vi "PicoScope6000aAdvancedTriggerDigital.vi"(0 "handle in":i16=16384, 2 "Digital Ports":T1 {"Digital Port  1"."Direction Channel 15" items=["Don't Care", "Low", "High", "Rising", "Falling"]; "Digital Port  1"."Direction Channel 14" items=["Don't Care", "Low", "High", "Rising", "Falling"]; "Digital Port  1"."Direction Channel 13" items=["Don't Care", "Low", "High", "Rising", "Falling"]; "Digital Port  1"."Direction Channel 12" items=["Don't Care", "Low", "High", "Rising", "Falling"]; "Digital Port  1"."Direction Channel 11" items=["Don't Care", "Low", "High", "Rising", "Falling"]; "Digital Port  1"."Direction Channel 10" items=["Don't Care", "Low", "High", "Rising", "Falling"]; "Digital Port  1"."Direction Channel 9" items=["Don't Care", "Low", "High", "Rising", "Falling"]; "Digital Port  1"."Direction Channel 8" items=["Don't Care", "Low", "High", "Rising", "Falling"]; "Digital Port  0"."Direction Channel 7" items=["Don't Care", "Low", "High", "Rising", "Falling"]; "Digital Port  0"."Direction Channel 6" items=["Don't Care", "Low", "High", "Rising", "Falling"]; "Digital Port  0"."Direction Channel 5" items=["Don't Care", "Low", "High", "Rising", "Falling"]; "Digital Port  0"."Direction Channel 4" items=["Don't Care", "Low", "High", "Rising", "Falling"]; "Digital Port  0"."Direction Channel 3" items=["Don't Care", "Low", "High", "Rising", "Falling"]; "Digital Port  0"."Direction Channel 2" items=["Don't Care", "Low", "High", "Rising", "Falling"]; "Digital Port  0"."Direction Channel 1" items=["Don't Care", "Low", "High", "Rising", "Falling"]; "Digital Port  0"."Direction Channel 0" items=["Don't Care", "Low", "High", "Rising", "Falling"]}, 11 "error in":errorcluster) -> (4 "handle out":i16=16384, 15 "error out":errorcluster)   [LabVIEW 2010]
doc: "This sub VI is an interface for the advanced trigger features of the oscilloscope to support digital channels."
uses:
  ps6000a.dll
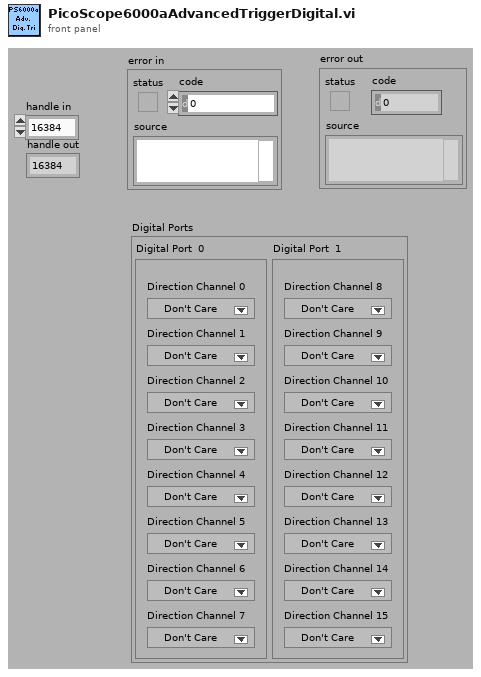
[diagram p1: front panel]
types:
  T1 = cluster{"Digital Port  0":cluster{"Direction Channel 0":u16, "Direction Channel 1":u16, "Direction Channel 2":u16, "Direction Channel 3":u16, "Direction Channel 4":u16, "Direction Channel 5":u16, "Direction Channel 6":u16, "Direction Channel 7":u16}, "Digital Port  1":cluster{"Direction Channel 8":u16, "Direction Channel 9":u16, "Direction Channel 10":u16, "Direction Channel 11":u16, "Direction Channel 12":u16, "Direction Channel 13":u16, "Direction Channel 14":u16, "Direction Channel 15":u16}}
  T2 = cluster{"Direction Channel 0":u16, "Direction Channel 1":u16, "Direction Channel 2":u16, "Direction Channel 3":u16, "Direction Channel 4":u16, "Direction Channel 5":u16, "Direction Channel 6":u16, "Direction Channel 7":u16}
  T3 = cluster{"Direction Channel 8":u16, "Direction Channel 9":u16, "Direction Channel 10":u16, "Direction Channel 11":u16, "Direction Channel 12":u16, "Direction Channel 13":u16, "Direction Channel 14":u16, "Direction Channel 15":u16}
  T4 = cluster{"status":bool, "code":u32, "source":string}
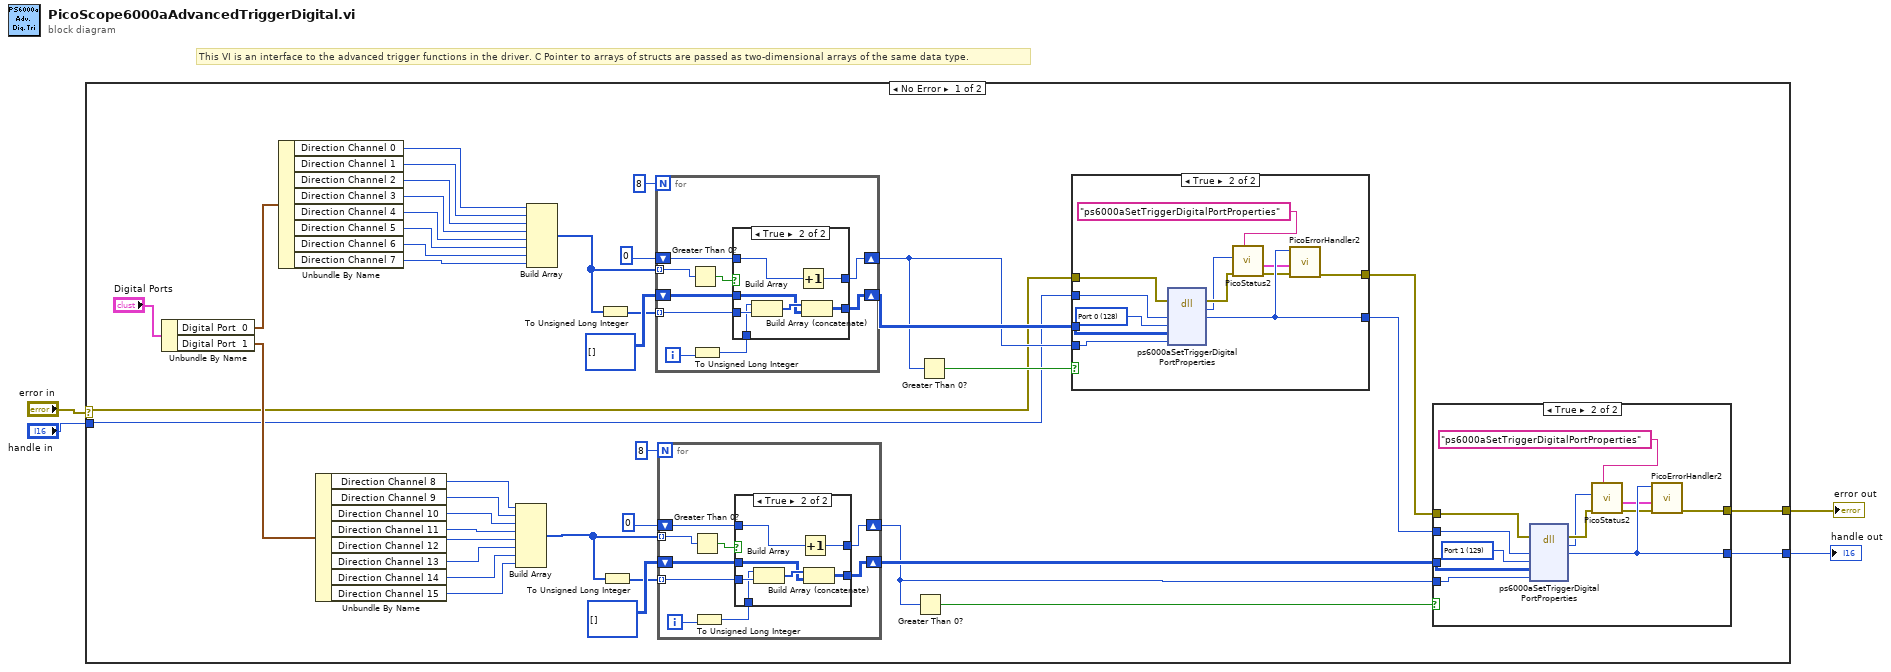
[diagram p0: block diagram]
diagram:
  # "This VI is an interface to the advanced trigger functions in the driver. C Pointer to arrays of structs are passed as two-dimensional arrays of the same data type."
  n1 = case shown="No Error" "error in" {
    selector: "error in" -> [w8 w110]
    tunnel: "handle in" -> [w7 w111]
    tunnel: [w5 w111] -> w2
    tunnel: [w6 w110] -> w1
    frame No Error {
      n2 = Unbundle By Name("Digital Ports") -> ("Digital Port  0"=w10:T2, "Digital Port  1"=w9:T3)
      n3 = Unbundle By Name(w10) -> ("Direction Channel 0"=w38:u16, "Direction Channel 1"=w45:u16, "Direction Channel 2"=w44:u16, "Direction Channel 3"=w43:u16, "Direction Channel 4"=w42:u16, "Direction Channel 5"=w41:u16, "Direction Channel 6"=w40:u16, "Direction Channel 7"=w39:u16)
      n4 = Unbundle By Name(w9) -> ("Direction Channel 8"=w20:u16, "Direction Channel 9"=w19:u16, "Direction Channel 10"=w13:u16, "Direction Channel 11"=w14:u16, "Direction Channel 12"=w15:u16, "Direction Channel 13"=w16:u16, "Direction Channel 14"=w17:u16, "Direction Channel 15"=w18:u16)
      n5 = Build Array(w20, w19, w13, w14, w15, w16, w17, w18) -> (w12:u16[])
      n6 = Build Array(w38, w45, w44, w43, w42, w41, w40, w39) -> (w33:u16[])
      n7 = To Unsigned Long Integer(number=w33) -> (unsigned 32bit integer=w34:u32[])
      n8 = To Unsigned Long Integer(number=w12) -> (unsigned 32bit integer=w21:u32[])
      n9 = for {
        N: 8 -> [_]
        tunnel: w34 -> [w98] mode=indexing
        shift-right: [w99] -> w30
        shift-left: i16 0 -> [w100]
        shift-right: [w96] -> w31
        shift-left: u32[][] [] -> [w97]
        tunnel: w33 -> [w94] mode=indexing
        i -> [w93]
        n10 = Greater Than 0?(x=w94) -> (x > 0?=w95:bool)
        n11 = To Unsigned Long Integer(number=w93) -> (unsigned 32bit integer=w92:u32)
        n12 = case shown="True" w95 {
          tunnel: w100 -> [w102 w109]
          tunnel: [w102 w106] -> w99
          tunnel: w98 -> [_ w108]
          tunnel: w92 -> [_ w107]
          tunnel: w97 -> [w101 w104]
          tunnel: [w101 w103] -> w96
          frame False {
          }
          frame True {
            n13 = Build Array(w107, w108) -> (w105:u32[])
            n14 = Increment(x=w109) -> (x+1=w106:i16)
            n15 = Build Array (concatenate)(w105, w104) -> (w103:u32[][])
          }
        }
      }
      n16 = for {
        N: 8 -> [_]
        tunnel: w21 -> [w52] mode=indexing
        shift-right: [w53] -> w26
        shift-left: i16 0 -> [w54]
        shift-right: [w50] -> w27
        shift-left: u32[][] [] -> [w51]
        tunnel: w12 -> [w48] mode=indexing
        i -> [w47]
        n17 = Greater Than 0?(x=w48) -> (x > 0?=w49:bool)
        n18 = To Unsigned Long Integer(number=w47) -> (unsigned 32bit integer=w46:u32)
        n19 = case shown="True" w49 {
          tunnel: w54 -> [w56 w63]
          tunnel: [w56 w60] -> w53
          tunnel: w52 -> [_ w62]
          tunnel: w46 -> [_ w61]
          tunnel: w51 -> [w55 w58]
          tunnel: [w55 w57] -> w50
          frame False {
          }
          frame True {
            n20 = Build Array(w61, w62) -> (w59:u32[])
            n21 = Increment(x=w63) -> (x+1=w60:i16)
            n22 = Build Array (concatenate)(w59, w58) -> (w57:u32[][])
          }
        }
      }
      n23 = Greater Than 0?(x=w26) -> (x > 0?=w25:bool)
      n24 = Greater Than 0?(x=w30) -> (x > 0?=w32:bool)
      n25 = case shown="True" w32 {
        tunnel: w7 -> [w78 w91]
        tunnel: w8 -> [w79 w90]
        tunnel: w30 -> [_ w89]
        tunnel: w31 -> [_ w88]
        tunnel: [w79 w86] -> w29
        tunnel: [w78 w87] -> w28
        frame False {
        }
        frame True {
          w85 = u32 128 items=["Port 0"=128, "Port 1"=129] ("Condition Action")
          n26 = dll-call lib="ps6000a.dll" fn="ps6000aSetTriggerDigitalPortProperties"(error in=w90, "handle"=w91, "Channel"=w85, "digitalDirections"=w88, "nDigitalDirections"=w89) -> (error out=w83:errorcluster, "PICO_STATUS"=w82:u32, "handle"=w87:i16)  [unwired: 5 in, 1 out]
          n27 = call "PicoStatus2.vi"("PICO source"="ps6000aSetTriggerDigitalPortProperties" ("source"), "Error in"=w83, "PICO STATUS"=w82) -> ("error out"=w84:errorcluster, "PICO_STATUS out"=w81:T4)  [unwired: 5 in]
          n28 = call "PicoErrorHandler2.vi"("error in (no error)"=w84, "PICO_STATUS in"=w81, "handle In"=w87) -> ("error out"=w86:errorcluster)  [unwired: 8 in]
        }
      }
      n29 = case shown="True" w25 {
        tunnel: w28 -> [w64 w77]
        tunnel: w29 -> [w65 w76]
        tunnel: w26 -> [_ w75]
        tunnel: w27 -> [_ w74]
        tunnel: [w65 w72] -> w6
        tunnel: [w64 w73] -> w5
        frame False {
        }
        frame True {
          w71 = u32 129 items=["Port 0"=128, "Port 1"=129] ("Condition Action")
          n30 = dll-call lib="ps6000a.dll" fn="ps6000aSetTriggerDigitalPortProperties"(error in=w76, "handle"=w77, "Channel"=w71, "digitalDirections"=w74, "nDigitalDirections"=w75) -> (error out=w69:errorcluster, "PICO_STATUS"=w67:u32, "handle"=w73:i16)  [unwired: 5 in, 1 out]
          n31 = call "PicoStatus2.vi"("PICO source"="ps6000aSetTriggerDigitalPortProperties" ("source"), "Error in"=w69, "PICO STATUS"=w67) -> ("error out"=w70:errorcluster, "PICO_STATUS out"=w68:T4)  [unwired: 5 in]
          n32 = call "PicoErrorHandler2.vi"("error in (no error)"=w70, "PICO_STATUS in"=w68, "handle In"=w73) -> ("error out"=w72:errorcluster)  [unwired: 8 in]
        }
      }
    }
    frame Error {
    }
  }
  "handle out" <- w2
  "error out" <- w1
